vi "New GPS Data Loop.vi"() -> ()   [LabVIEW 2011]
uses:
  <instrlib>/NavCom SF-2050/NavCom SF-2050.lvlib
panel:
  in  "stop?":bool
  out "NMEA String":string
  in  "error in (no error)":errorcluster
  out "error out":errorcluster
  in  "Debug":bool
  in  "VISA resource name":refnum<visa-resource-name>
  in  "Serial Configuration":cluster{"Baud Rate":u32, "Parity":u16}={"Baud Rate"=115200, "Parity"=0} {"Parity" items=["None", "Odd", "Even", "Mark", "Space"]; "Baud Rate" items=["1200"=1200, "2400"=2400, "4800"=4800, "9600"=9600, "19200"=19200, "38400"=38400, "57600"=57600, "115200"=115200]}
  out "GPS Data":T1 {"Time"."GPS Time of Week" format="%.3f"; "Velocity, Correction & SET"."Extended Navigation Mode" items=["Non Differential"=0, "Code (RTCM Type 1 & 9)"=1, "Code, Single Frequency (WAAS)"=2, "Code, Dual Frequency (WAAS)"=3, "Code, Single Frequency (WCT)"=4, "Code/RCP, Dual Frequency (WCT)"=5, "Code, Single Frequency (RTG)"=6, "Code (RTCM Type 1 & 9) Dual Frequency"=10, "Code/RCP, Dual Frequency (RTG)"=11, "Code, Single Frequency (NCT-RTK)"=12, "Code, Single Frequency (RTCM 18 & 19)"=13, "Code, Single Frequency (RTCM 21 & 22)"=14, "Code, Single Frequency (CMR)"=15, "Code, Dual Frequency (NCT-RTK)"=16, "Code, Dual Frequency (RTCM 18 & 19)"=17, "Code, Dual Frequency (RTCM 20 & 21)"=18, "Code, Dual Frequency (CMR)"=19, "RTK (NCT-RTK)"=20, "RTK (RTCM 18 & 19)"=21, "RTK (RTCM 20 & 21)"=22, "RTK (CMR)"=23, "Code, Single Frequency with SET (RTG)"=24, "Code/RCP, Dual Frequency with SET (RTG)"=25, "RTK Extend"=26]; "Altitude" format="%#_18g"; "Longitude" format="%#_18g"; "Latitude" format="%#_18g"}
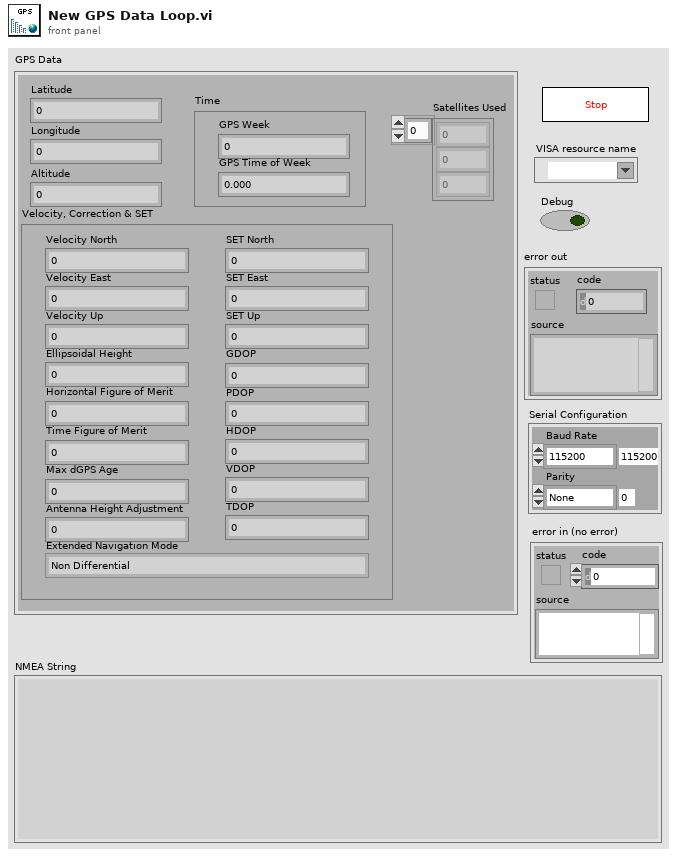
[diagram p1: front panel]
types:
  T1 = cluster{"Latitude":dbl, "Longitude":dbl, "Altitude":dbl, "Velocity, Correction & SET":cluster{"Velocity North":dbl, "Velocity East":dbl, "Velocity Up":dbl, "Ellipsoidal Height":dbl, "GDOP":sgl, "PDOP":sgl, "HDOP":sgl, "VDOP":sgl, "TDOP":sgl, "Horizontal Figure of Merit":u8, "Time Figure of Merit":u8, "Max dGPS Age":sgl, "Extended Navigation Mode":u8, "Antenna Height Adjustment ":dbl, "SET North":i32, "SET East":i32, "SET Up":i32}, "Time":cluster{"GPS Week":u16, "GPS Time of Week":sgl}, "Satellites Used":i32[]}
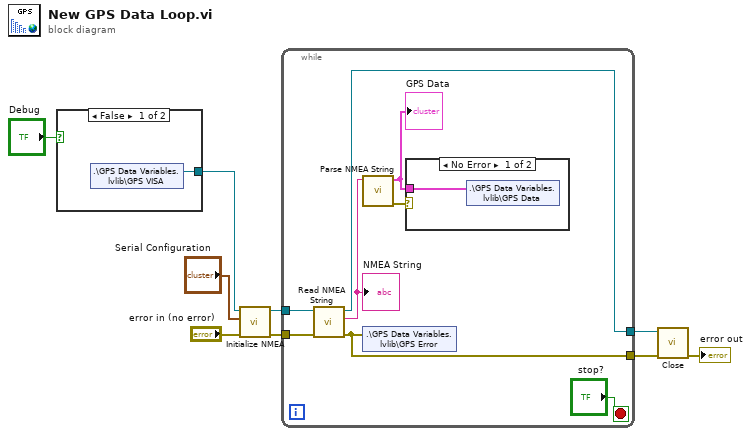
[diagram p0: block diagram]
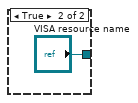
[diagram p2: hidden frame]
diagram:
  n1 = case shown="False" "Debug" {
    tunnel: [w10 "VISA resource name"] -> w3
    frame False {
      n2 = shared-variable ".\\GPS Data Variables.lvlib\\GPS VISA"() -> (w10:refnum<visa-resource-name>)  [unwired: 1 in, 1 out]
    }
    frame True {
    }
  }
  n3 = call <instrlib>:"Initialize NMEA.vi"("error in (no error)"="error in (no error)", "Serial Configuration"="Serial Configuration", "VISA resource name"=w3) -> ("error out"=w7:errorcluster, "VISA resource name out"=w8:refnum<visa-resource-name>)  [unwired: 7 in]
  n4 = while {
    tunnel: w7 -> [w18]
    tunnel: w8 -> [w19]
    tunnel: [w17] -> w6
    tunnel: [w16] -> w5
    stop <- "stop?" stop-if-true
    n5 = call <instrlib>:"Read NMEA String.vi"("error in (no error)"=w18, "VISA resource name"=w19) -> ("error out"=w16:errorcluster, "NMEA String"=w15:string, "VISA resource name out"=w17:refnum<visa-resource-name>)  [unwired: 7 in]
    "NMEA String" <- w15
    n6 = call "Parse NMEA String.vi"("NMEA String"=w15) -> ("Error Out"=w13:errorcluster, "GPS Data Out"=w12:T1)  [unwired: 9 in]
    "GPS Data" <- w12
    n7 = shared-variable ".\\GPS Data Variables.lvlib\\GPS Error"(w16) -> ()  [unwired: 1 in, 1 out]
    n8 = case shown="No Error" w13 {
      tunnel: w12 -> [w20 _]
      frame No Error {
        n9 = shared-variable ".\\GPS Data Variables.lvlib\\GPS Data"(w20) -> ()  [unwired: 1 in, 1 out]
      }
      frame Error {
      }
    }
  }
  n10 = call <instrlib>:"Close.vi"("error in (no error)"=w5, "VISA resource name"=w6) -> ("error out"=→"error out":errorcluster)  [unwired: 9 in]
